vi "SWAT-TSM record.vi"() -> ()   [LabVIEW 2020]
uses:
  <vilib>/Instr/_visa.llb/VISA Configure Serial Port (Instr).vi
panel:
  out "$PGSI2 sentence":string
  in  "*.txt Path":path
  out "String":string
  in  "baud rate (9600)":u32=9600
  in  "COM Port":refnum<visa-resource-name>
  in  "Stop":bool
  in  "Start":bool
  # "Records data from SWAT-TSM ECU / Rel.V. 2022.1"
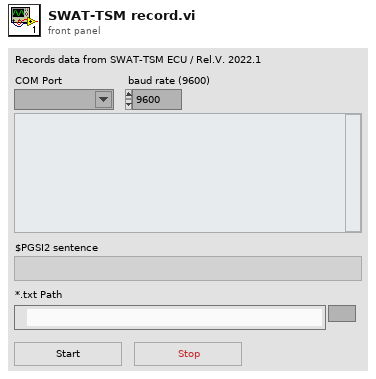
[diagram p1: front panel]
types:
  T1 = enum16{"open", "replace", "create", "open or create", "replace or create", "replace or create with confirmation"}
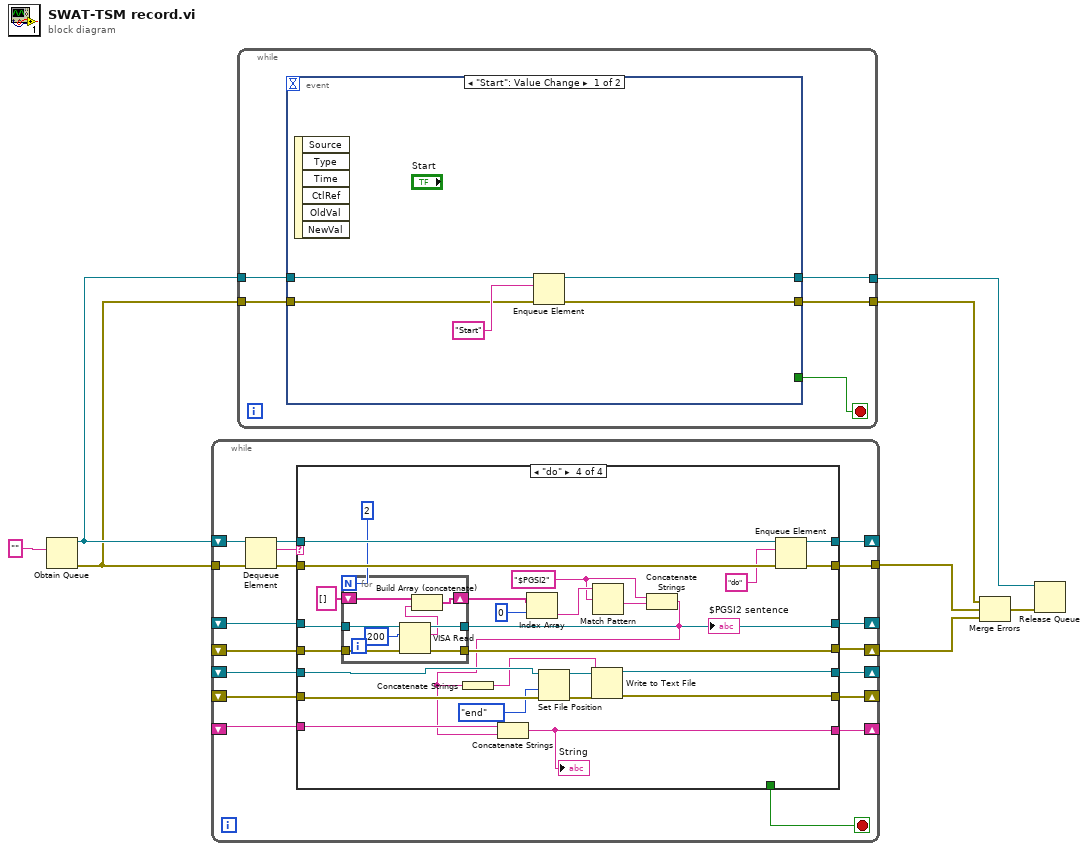
[diagram p0: block diagram]
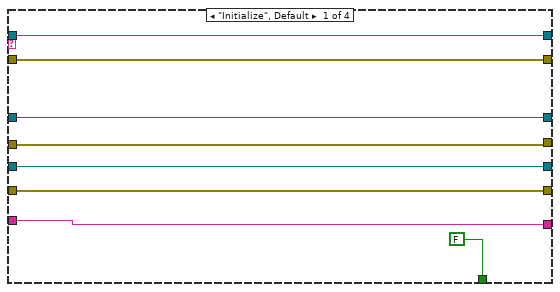
[diagram p2: hidden frame]
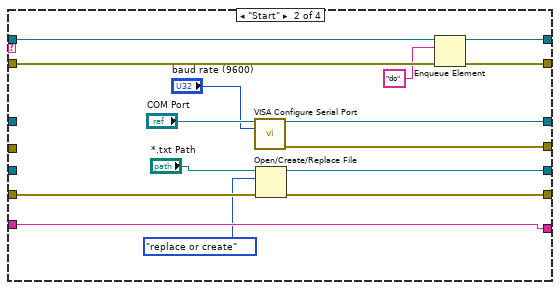
[diagram p3: hidden frame]
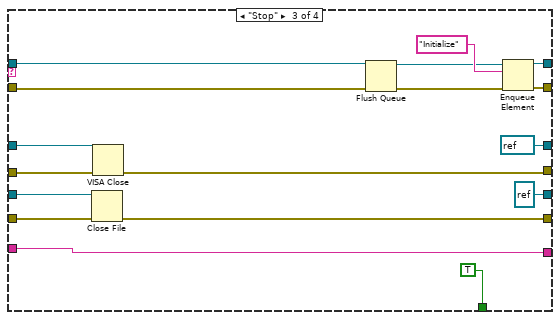
[diagram p4: hidden frame]
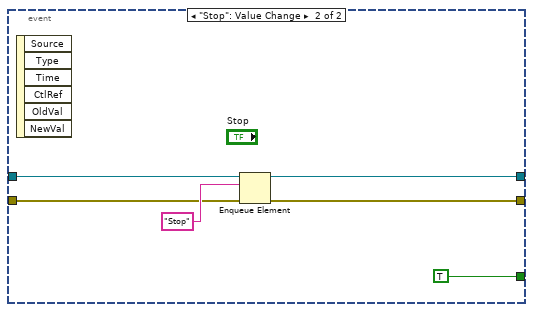
[diagram p5: hidden frame]
diagram:
  n1 = Obtain Queue(element data type="") -> (queue out=w8:refnum<queue>, error out=w6:errorcluster)  [unwired: 4 in, 1 out]
  n2 = while {
    shift-right: [w24] -> _
    shift-left: _ -> [w22]
    shift-right: [w23] -> w5
    shift-left: _ -> [w21]
    tunnel: [w17] -> w4
    shift-right: [w18] -> _
    shift-left: w8 -> [w26]
    tunnel: w6 -> [w16]
    shift-right: [w13] -> _
    shift-left: _ -> [w14]
    shift-right: [w11] -> _
    shift-left: _ -> [w10]
    shift-right: [w12] -> _
    shift-left: _ -> [w9]
    stop <- w15 stop-if-true
    n3 = Dequeue Element(queue=w26, error in (no error)=w16) -> (queue out=w20:refnum<queue>, element=w25:string, error out=w19:errorcluster)  [unwired: 1 in, 1 out]
    n4 = case shown="\"do\"" w25 {
      tunnel: [w32 w47 refnum<visa-resource-name> refnum ("VISA resource name out") w86] -> w24
      tunnel: [w31 w46 w61 w85] -> w23
      tunnel: w22 -> [w32 _ w62 w87]
      tunnel: w21 -> [w31 _ w63 w88]
      tunnel: w20 -> [w34 w44 w55 w93]
      tunnel: w19 -> [w33 w45 w56 w92]
      tunnel: [w34 w43 w66 w91] -> w18
      tunnel: [w33 w42 w65 w90] -> w17
      tunnel: [FALSE _ TRUE _] -> w15
      tunnel: w14 -> [w29 w40 w54 w84]
      tunnel: [w29 w40 w54 w83] -> w13
      tunnel: [w28 w39 refnum<file> refnum ("refnum out") w81] -> w12
      tunnel: [w27 w38 w51 w82] -> w11
      tunnel: w10 -> [w27 w37 w53 w77]
      tunnel: w9 -> [w28 _ w52 w80]
      frame "Initialize", Default {
      }
      frame "Start" {
        n5 = call-poly "VISA Configure Serial Port"("VISA resource name"="COM Port", "baud rate (9600)"="baud rate (9600)") -> ("VISA resource name out"=w47:refnum<visa-resource-name>, "error out"=w46:errorcluster)  [unwired: 12 in]
        n6 = Open/Create/Replace File(file path (use dialog)="*.txt Path", error in=w37, operation (0:open)=T1."replace or create") -> (refnum out=w39:refnum<file>, error out=w38:errorcluster)  [unwired: 3 in, 1 out]
        n7 = Enqueue Element(queue=w44, element="do", error in (no error)=w45) -> (queue out=w43:refnum<queue>, error out=w42:errorcluster)  [unwired: 1 in, 1 out]
      }
      frame "Stop" {
        n8 = Close File(refnum=w52, error in=w53) -> (error out=w51:errorcluster)  [unwired: 1 out]
        n9 = VISA Close(VISA resource name=w62, error in (no error)=w63) -> (error out=w61:errorcluster)
        n10 = Flush Queue(queue=w55, error in (no error)=w56) -> (queue out=w58:refnum<queue>, error out=w57:errorcluster)  [unwired: 1 out]
        n11 = Enqueue Element(queue=w58, element="Initialize", error in (no error)=w57) -> (queue out=w66:refnum<queue>, error out=w65:errorcluster)  [unwired: 1 in, 1 out]
      }
      frame "do" {
        w68 = "$PGSI2"
        n12 = for {
          N: 2 -> [_]
          tunnel: w88 -> [w101]
          tunnel: w87 -> [w100]
          tunnel: [w98] -> w86
          tunnel: [w97] -> w85
          shift-right: [w96] -> w72
          shift-left: string[] [] -> [w95]
          n13 = VISA Read(VISA resource name=w100, byte count=200, error in (no error)=w101) -> (VISA resource name out=w98:refnum<visa-resource-name>, read buffer=w94:string, error out=w97:errorcluster)  [unwired: 1 out]
          n14 = Build Array (concatenate)(w95, w94) -> (w96:string[])
        }
        n15 = Index Array(array=w72, index=0) -> (element=w70:string)
        n16 = Set File Position(refnum=w80, from (0:start)=enum16{"start", "end", "current"}."end", error in=w77) -> (refnum out=w79:refnum<file>, error out=w78:errorcluster)  [unwired: 1 in]
        n17 = Match Pattern(string=w70, regular expression=w68) -> (after substring=w69:string)  [unwired: 1 in, 3 out]
        n18 = Concatenate Strings(w68, w69) -> (w67:string)
        "$PGSI2 sentence" <- w67
        n19 = Concatenate Strings(w67) -> (w74:string)
        n20 = Concatenate Strings(w84, w67) -> (w83:string)
        "String" <- w83
        n21 = Write to Text File(file (use dialog)=w79, text=w74, error in=w78) -> (refnum out=w81:refnum<file>, error out=w82:errorcluster)  [unwired: 1 in, 1 out]
        n22 = Enqueue Element(queue=w93, element="do", error in (no error)=w92) -> (queue out=w91:refnum<queue>, error out=w90:errorcluster)  [unwired: 1 in, 1 out]
      }
    }
  }
  n23 = while {
    tunnel: w8 -> [w106]
    tunnel: [w105] -> w1
    tunnel: w6 -> [w104]
    tunnel: [w103] -> w3
    stop <- w102 stop-if-true
    n24 = event shown="[0] \"Start\": Value Change" {
      selector: _ -> [_ _]
      dyn-events: _ -> [_ _]
      timeout: _ -> [_ _]
      tunnel: w106 -> [w111 w117]
      tunnel: [w110 w115] -> w105
      tunnel: w104 -> [w108 w113]
      tunnel: [w107 w112] -> w103
      tunnel: [_ TRUE] -> w102
      event "Start": Value Change {
        n25 = event-data() -> ()  [unwired: 1 in, 6 out]
        n26 = Enqueue Element(queue=w111, element="Start", error in (no error)=w108) -> (queue out=w110:refnum<queue>, error out=w107:errorcluster)  [unwired: 1 in, 1 out]
      }
      event "Stop": Value Change {
        n27 = event-data() -> ()  [unwired: 1 in, 6 out]
        n28 = Enqueue Element(queue=w117, element="Stop", error in (no error)=w113) -> (queue out=w115:refnum<queue>, error out=w112:errorcluster)  [unwired: 1 in, 1 out]
      }
    }
  }
  n29 = Merge Errors(w3, w4, w5) -> (w2:errorcluster)
  n30 = Release Queue(queue=w1, error in (no error)=w2) -> ()  [unwired: 1 in, 3 out]
